vi "Normal String to Hex String.vi"(11 "Command Opcode":string) -> (3 "Hex String":string)   [LabVIEW 2020]
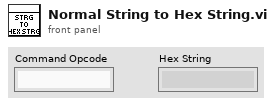
[diagram p1: front panel]
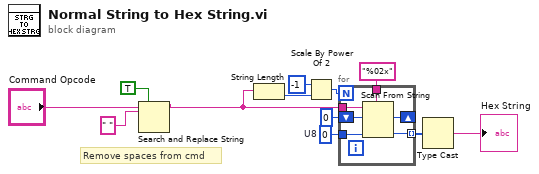
[diagram p0: block diagram]
diagram:
  w6 = u8 0  # U8
  # "Remove spaces from cmd"
  n1 = Search and Replace String(replace all?=TRUE ("replace all? (F)"), input string="Command Opcode", search string=" ") -> (result string=w2:string)  [unwired: 5 in, 3 out]
  n2 = String Length(string=w2) -> (length=w9:i32)
  n3 = Scale By Power Of 2(n=-1, x=w9) -> (x*2^n=w11:i32)
  n4 = for {
    N: w11 -> [_]
    shift-right: [w17] -> _
    shift-left: u32 0 -> [w18]
    tunnel: w2 -> [w16]
    tunnel: w6 -> [w15]
    tunnel: [w14] -> w7 mode=indexing
    tunnel: "%02x" ("format string") -> [w13]
    n5 = Scan From String(format string=w13, input string=w16, initial scan location=w18, default 1=w15) -> (offset past scan=w17:u32, output 1=w14:u8)  [unwired: 1 in, 2 out]
  }
  n6 = Type Cast(x=w7) -> (*(type *) &x=→"Hex String":string)  [unwired: 1 in]
